vi "test.vi"(8 "error in (no error)":errorcluster) -> (0 "error out":errorcluster, 3 "Full Report":string)   [LabVIEW 2019, in "labview_json_tests.lvlib"]
uses:
  labview_json_tests.lvlib
panel:
  out "ms Avg Dump":dbl
  out "ms Avg Load":dbl
  in  "Show Passed? (F)":bool
  out "All Passed?":bool
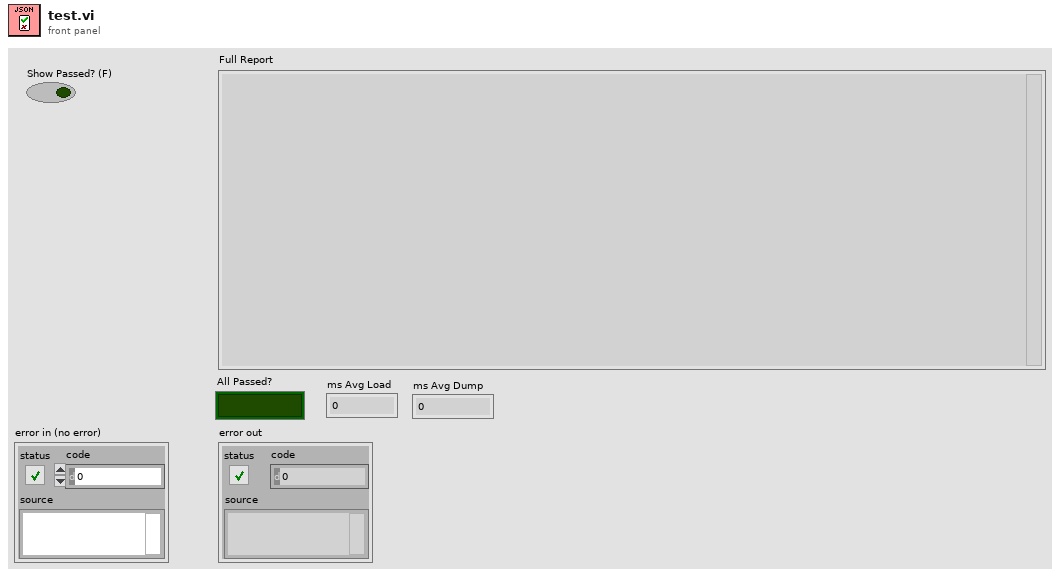
[diagram p1: front panel]
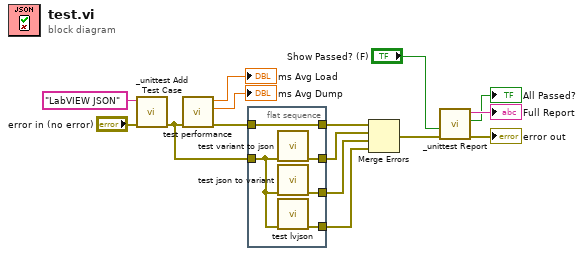
[diagram p0: block diagram]
diagram:
  n1 = call "_unittest Add Test Case.vi"("error in (no error)"="error in (no error)", "Test Case"="LabVIEW JSON") -> ("error out"=w5:errorcluster)  [unwired: 9 in]
  n2 = call "test performance.vi"("error in (no error)"=w5) -> ("error out"=w4:errorcluster, "ms Avg Dump"=→"ms Avg Dump":dbl, "ms Avg Load"=→"ms Avg Load":dbl)  [unwired: 8 in]
  n3 = flat-sequence {
    tunnel: [w20] -> w10
    tunnel: [w19] -> w9
    tunnel: [w18] -> w6
    tunnel: w5 -> [w17]
    tunnel: [w16] -> w3
    tunnel: w4 -> [w16]
    frame #0 {
      n4 = call "test variant to json.vi"("error in (no error)"=w17) -> ("error out"=w20:errorcluster)  [unwired: 10 in]
      n5 = call "test json to variant.vi"("error in (no error)"=w17) -> ("error out"=w19:errorcluster)  [unwired: 10 in]
      n6 = call "test lvjson.vi"("error in (no error)"=w17) -> ("error out"=w18:errorcluster)  [unwired: 10 in]
    }
  }
  n7 = Merge Errors(w3, w10, w9, w6) -> (w13:errorcluster)
  n8 = call "_unittest Report.vi"("error in (no error)"=w13, "Show Passed? (F)"="Show Passed? (F)") -> ("error out"=→"error out":errorcluster, "All Passed?"=→"All Passed?":bool, "Full Report"=→"Full Report":string)  [unwired: 7 in]
